vi "Main.vi"() -> ()   [LabVIEW 2017]
uses:
  <vilib>/myRIO/Common/Instrument Driver Framework/myRIO v1.0/UART/vis/myRIO v1.0 Close UART.vi
  <vilib>/myRIO/Common/Instrument Driver Framework/myRIO v1.0/PWM/vis/myRIO v1.1 Open PWM.vi
  <vilib>/myRIO/Common/Instrument Driver Framework/Utilities/vis/Validate Channels.vi
  <vilib>/myRIO/Common/Instrument Driver Framework/myRIO v1.0/PWM/vis/myRIO v1.0 Reserve PWM.vi
  <vilib>/myRIO/Common/Instrument Driver Framework/myRIO v1.0/PWM/vis/myRIO v1.0 Build MUX Configuration PWM.vi
  <vilib>/myRIO/Common/Instrument Driver Framework/myRIO v1.0/Resource Manager/vis/myRIO v1.0 Reserve Channel List.vi
  <vilib>/myRIO/Common/Instrument Driver Framework/myRIO v1.0/Resource Manager/vis/myRIO v1.0 Create Configuration List.vi
  <vilib>/myRIO/Common/Instrument Driver Framework/myRIO v1.0/Resource Manager/vis/myRIO v1.0 Reserve Channel.vi
  <vilib>/myRIO/Common/Instrument Driver Framework/myRIO v1.0/Resource Manager/vis/myRIO v1.0 Unreserve Channel.vi
  <vilib>/myRIO/Common/Instrument Driver Framework/myRIO v1.0/Resource Manager/vis/myRIO v1.0 Build Mutex Name.vi
  <vilib>/Utility/VariantDataType/GetNumericInfo.vi
  <vilib>/Utility/error.llb/Error Cluster From Error Code.vi
  <vilib>/myRIO/Common/Instrument Driver Framework/myRIO v1.0/myRIO v1.1 Open.vi
  <vilib>/myRIO/Common/Instrument Driver Framework/Utilities/vis/IO Manager.vi
  <vilib>/myRIO/Common/Instrument Driver Framework/Utilities/vis/Configuration Manager.vi
  <vilib>/myRIO/Common/Instrument Driver Framework/myRIO v1.0/Resource Manager/vis/myRIO v1.0 Configure IO.vi
  <vilib>/myRIO/Common/Instrument Driver Framework/myRIO v1.0/myRIO v1.0 Close.vi
  <vilib>/myRIO/Common/Instrument Driver Framework/Utilities/vis/FPGA Ref Manager.vi
  <vilib>/myRIO/Common/Instrument Driver Framework/myRIO v1.0/myRIO v1.0 Reset FPGA.vi
  <vilib>/myRIO/Common/Instrument Driver Framework/myRIO v1.0/IRQ/vis/myRIO v1.0 IRQ Info FGV.vi
  <vilib>/myRIO/Common/Instrument Driver Framework/myRIO v1.0/IRQ/vis/myRIO v1.0 Timer IRQ Info FGV.vi
  <vilib>/myRIO/Common/Instrument Driver Framework/myRIO v1.0/IRQ/vis/myRIO v1.0 ISR Agent.vi
  <vilib>/myRIO/Instrument Drivers/Utilities/Utilities.lvlib
  <vilib>/myRIO/Instrument Drivers/Onboard IO/PWM/PWM.lvlib
panel:
  out "position [%FS] 6":dbl
  out "position [%FS] 2":dbl
  out "position [%FS]":dbl
  out "Numeric 4":dbl
  out "Numeric 3":dbl
  out "Numeric 2":dbl
  in  "position [%FS] 5":dbl(slide) scale=-200.0..200.0
  in  "freq [Hz] 5":dbl=50.0
  out "pulse width [ms] 5":dbl=1.5
  out "duty cycle [%] 5":dbl
  in  "null offset 5":bool
  out "offset [%FS] 5":dbl
  in  "position [%FS] 4":dbl(slide) scale=-200.0..200.0
  in  "freq [Hz] 4":dbl=50.0
  out "pulse width [ms] 4":dbl=1.5
  out "duty cycle [%] 4":dbl
  in  "null offset 4":bool
  out "offset [%FS] 4":dbl
  in  "PWM channel 3":tag="B/PWM0"
  in  "position [%FS] 3":dbl(slide) scale=-200.0..200.0
  in  "freq [Hz] 3":dbl=50.0
  out "pulse width [ms] 3":dbl=1.5
  out "duty cycle [%] 3":dbl
  in  "null offset 3":bool
  out "offset [%FS] 3":dbl
  in  "PWM channel 2":tag="B/PWM0"
  in  "PWM channel":tag="B/PWM0"
  in  "[ESC]":bool
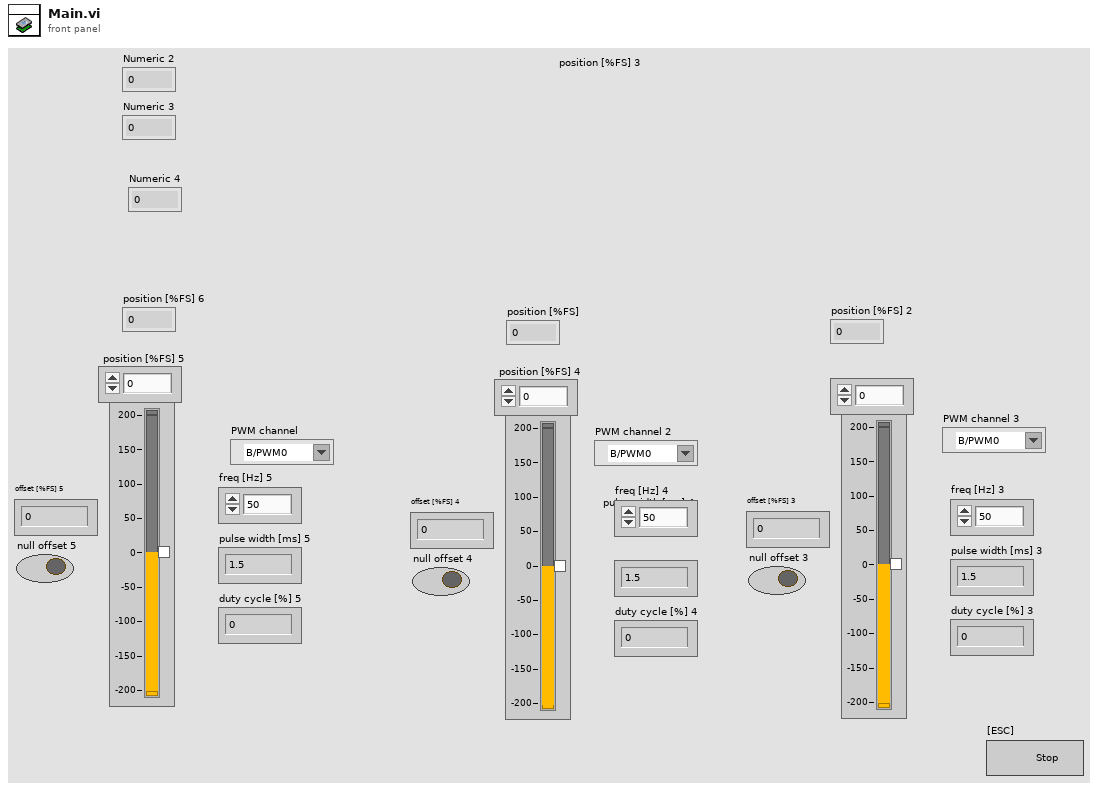
[diagram p1: front panel]
types:
  T1 = enum16{"", "INICIO", "STOP", "DETECCION", "ESPERA", "MOVIMIENTO"}
  T2 = typedef "PWM.lvlib/PWM Reference.ctl" = cluster{"myRIO Reference":T3, "PWM Channels Enum":T7, "PWM Configuration":T8}
  T3 = typedef "myRIO Generic Hardware Reference.ctl" = cluster{"myRIO Model":T4, "myRIO Hardware Reference":T5}
  T4 = typedef "Hardware Version Enum.ctl" = enum16{"Unknown", "myRIO-1900", "myRIO-1950", "roboRIO", "NI ELVIS RIO CM"}
  T5 = typedef "myRIO v1.0 Reference.ctl" = cluster{"Generic FPGA Reference":T6, "Allow multiple opens":bool}
  T6 = typedef "Generic FPGA Reference.ctl" = refnum<k20>
  T7 = typedef "PWM Channels Enum.ctl" = enum16{"Not Connected", "C/PWM0", "C/PWM1", "A/PWM0", "A/PWM1", "A/PWM2", "B/PWM0", "B/PWM1", "B/PWM2", "PWM/PWM0", "PWM/PWM1", "PWM/PWM2", "PWM/PWM3", "PWM/PWM4", "PWM/PWM5", "PWM/PWM6", "PWM/PWM7", "PWM/PWM8", "PWM/PWM9"}
  T8 = typedef "PWM.lvlib/PWM Configuration.ctl" = cluster{"Frequency":dbl, "Duty Cycle":dbl}
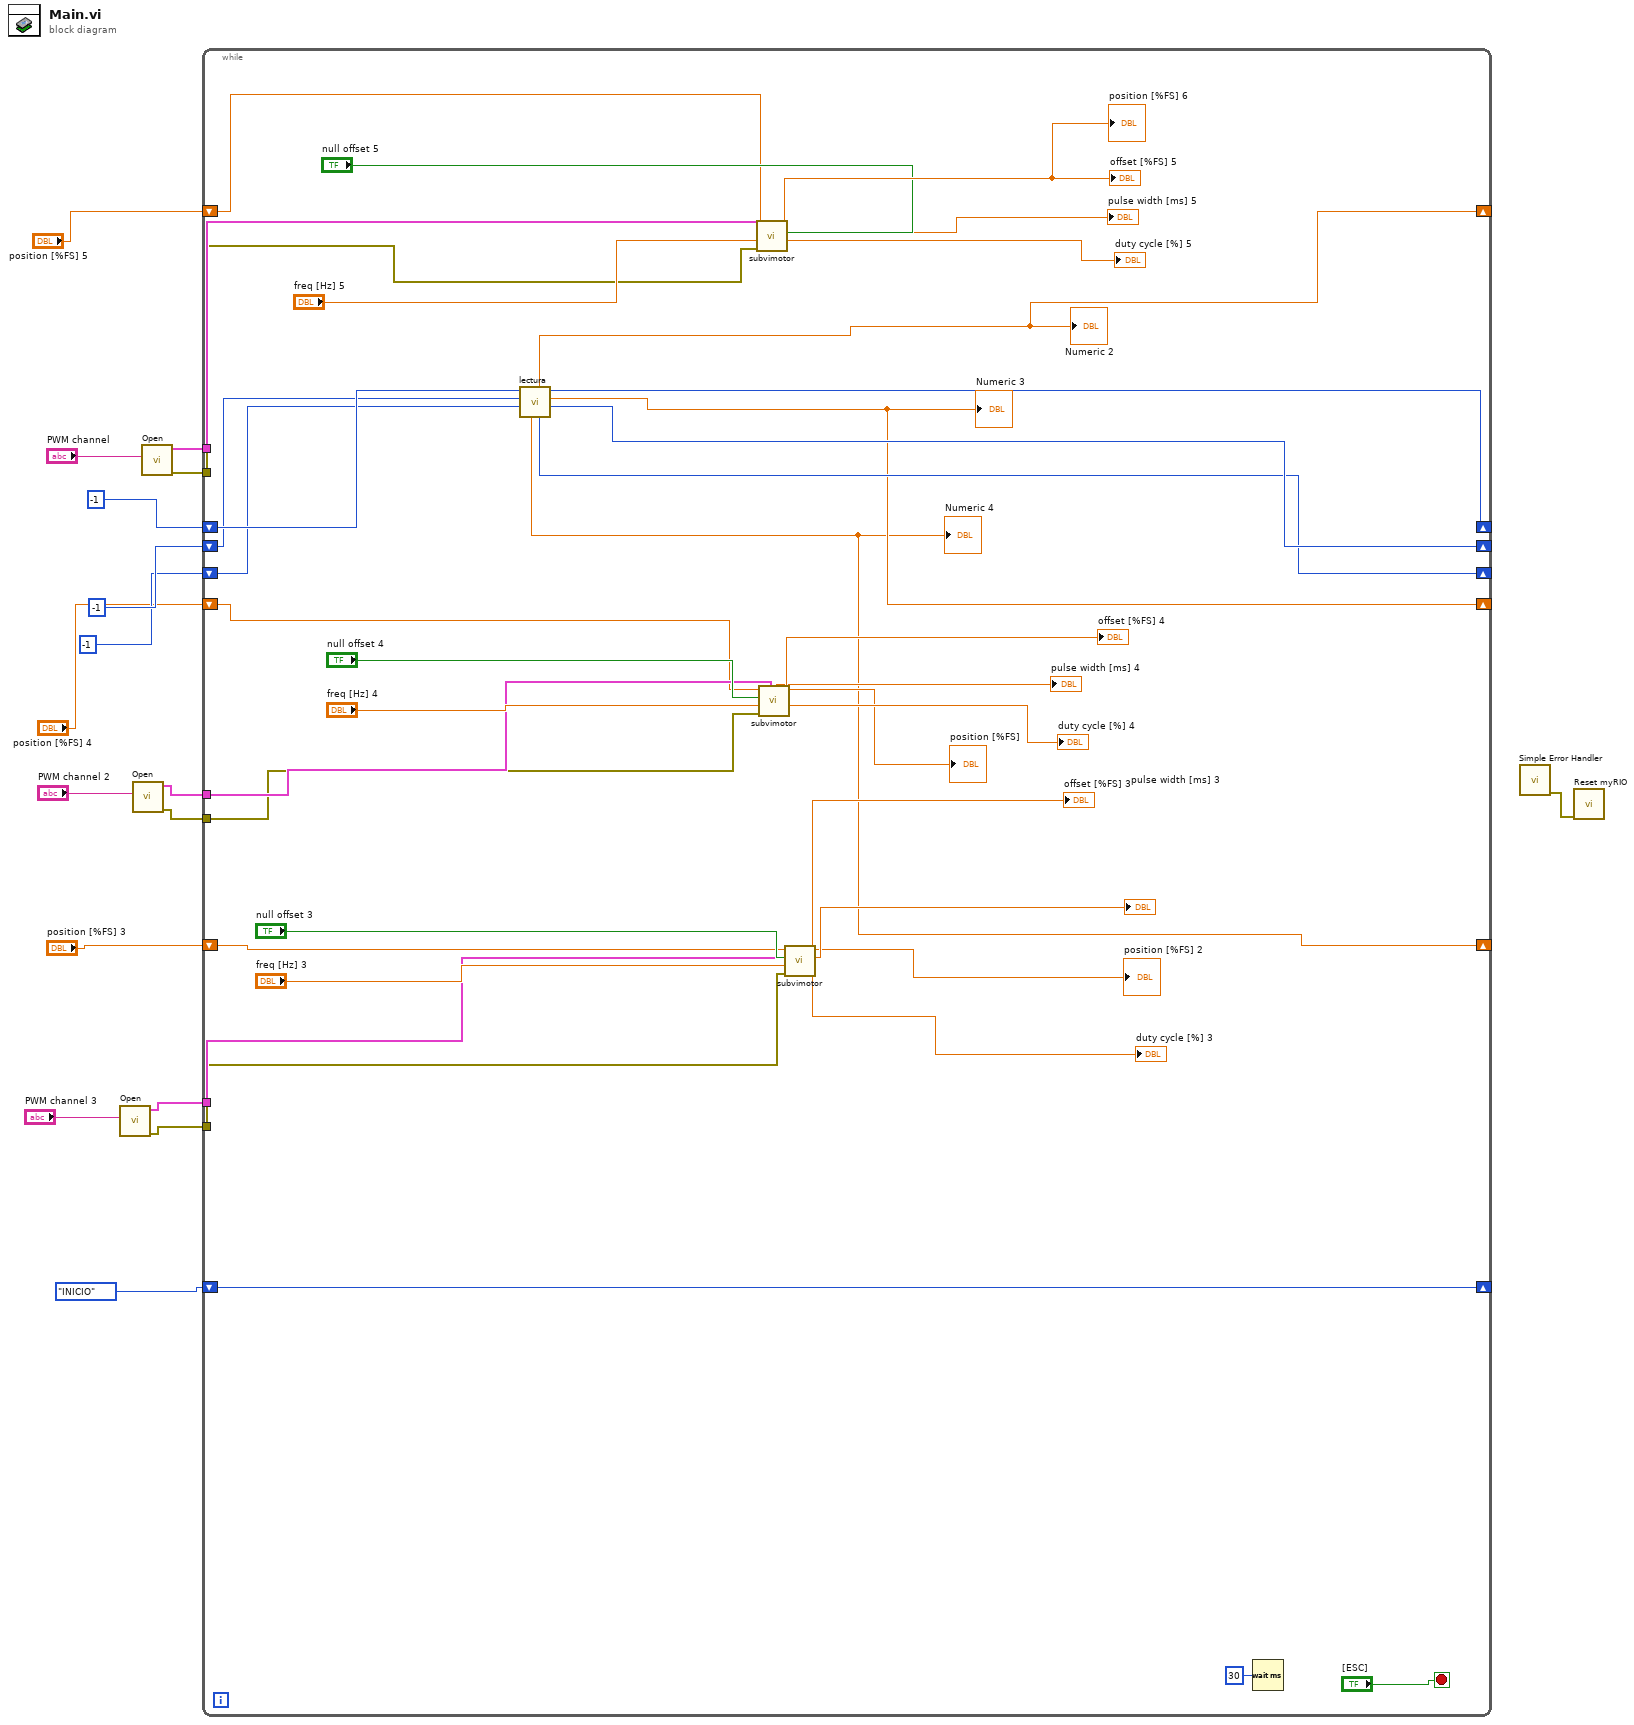
[diagram p0: block diagram]
diagram:
  n1 = call <vilib>:"Open.vi"("Channel Name"="PWM channel 3") -> ("error out"=w8:errorcluster, "PWM Ref Out"=w9:T2)  [unwired: 9 in]
  n2 = call <vilib>:"Open.vi"("Channel Name"="PWM channel 2") -> ("error out"=w11:errorcluster, "PWM Ref Out"=w12:T2)  [unwired: 9 in]
  n3 = call <vilib>:"Open.vi"("Channel Name"="PWM channel") -> ("error out"=w14:errorcluster, "PWM Ref Out"=w15:T2)  [unwired: 9 in]
  n4 = while {
    tunnel: w15 -> [w33]
    tunnel: w14 -> [w32]
    tunnel: w12 -> [w40]
    tunnel: w11 -> [w39]
    tunnel: w9 -> [w47]
    tunnel: w8 -> [w46]
    shift-right: [w25] -> _
    shift-left: -1 -> [w30]
    shift-right: [w29] -> _
    shift-left: -1 -> [w28]
    shift-right: [w27] -> _
    shift-left: -1 -> [w26]
    shift-right: [w24] -> _
    shift-left: "position [%FS] 5" -> [w23]
    shift-right: [w22] -> _
    shift-left: "position [%FS] 4" -> [w21]
    shift-right: [w20] -> _
    shift-left: "position [%FS] 3" -> [w19]
    shift-right: [w18] -> _
    shift-left: T1."INICIO" -> [w18]
    stop <- "[ESC]" stop-if-true
    n5 = call "lectura.vi"("Numeric in"=w26, "Numeric 3"=w28, "entrada1"=w30) -> ("Numeric 4"=w29:i32, "Real Matrix Element 2"=w22:dbl, "salida1"=w25:i32, "Numeric out"=w27:i32, "Real Matrix Element 3"=w24:dbl, "Real Matrix Element"=w20:dbl)  [unwired: 3 in]
    "Numeric 2" <- w24
    "Numeric 3" <- w22
    "Numeric 4" <- w20
    n6 = call "subvimotor.vi"("PWM Ref Out"=w33, "error in (no error)"=w32, "freq [Hz] 3"="freq [Hz] 5", "null offset 3"="null offset 5", "position [%FS] 3"=w23) -> ("Numeric"=→"duty cycle [%] 5":dbl, "Numeric 2"=→"pulse width [ms] 5":dbl, "position [%FS]"=→"offset [%FS] 5" →"position [%FS] 6":dbl)  [unwired: 4 in]
    n7 = call "subvimotor.vi"("PWM Ref Out"=w40, "error in (no error)"=w39, "freq [Hz] 3"="freq [Hz] 4", "null offset 3"="null offset 4", "position [%FS] 3"=w21) -> ("Numeric"=→"duty cycle [%] 4":dbl, "Numeric 2"=→"pulse width [ms] 4":dbl, "position [%FS]"=→"offset [%FS] 4" →"position [%FS]":dbl)  [unwired: 4 in]
    n8 = call "subvimotor.vi"("PWM Ref Out"=w47, "error in (no error)"=w46, "freq [Hz] 3"="freq [Hz] 3", "null offset 3"="null offset 3", "position [%FS] 3"=w19) -> ("Numeric"=→"duty cycle [%] 3":dbl, "Numeric 2"=→"pulse width [ms] 3":dbl, "position [%FS]"=→"offset [%FS] 3" →"position [%FS] 2":dbl)  [unwired: 4 in]
    n9 = Wait (ms)(milliseconds to wait=u32 30) -> ()  [unwired: 1 out]
  }
  n10 = call <vilib>:"Simple Error Handler.vi"() -> ("error out"=w17:errorcluster)  [unwired: 5 in, 4 out]
  n11 = call <vilib>:"Reset myRIO.vi"("error in (no error)"=w17) -> ()  [unwired: 10 in, 1 out]
